vi "Real_Time_Main.vi"() -> ()   [LabVIEW 2020]
uses:
  control/uart_data.ctl
  control/logging_data.ctl
  control/system_monitoring_data.ctl
  Host/control/host_data.ctl
  <vilib>/Analysis/baseanly.llb/Mean (DBL).vi
  ae3b70e6-cfa7-4b88-a663-fdf942523340.vi
  <vilib>/Instr/_visa.llb/VISA Configure Serial Port (Instr).vi
  <vilib>/FPGAPlugInAG/cRIO-9030/niLvFpga_Open_cRIO-9030.vi
  <vilib>/rvi/interface/common/dynamic/niFpgaDynamicAddResources.vi
  <vilib>/FPGAPlugInAG/Dynamic/niLvFpga_Reset_Dynamic.vi
  <vilib>/FPGAPlugInAG/Dynamic/niLvFpga_Run_Dynamic.vi
  <vilib>/Utility/error.llb/Error Cluster From Error Code.vi
  <vilib>/rvi/errors/niLvFpgaAdjustHostInterfaceError.vi
  <vilib>/FPGAPlugInAG/Dynamic/niLvFpga_Close_Dynamic.vi
  <vilib>/rvi/interface/nirviOpenFPGA/nirviOpenFPGA.xnode
  FPGA/build/excavatorsimulat_FPGATarget_FPGAMain_YO9VNoECHsQ.lvbitx
  <vilib>/rvi/interface/nirviMethod/nirviMethod.xnode
  <vilib>/rvi/interface/nirviReadWriteControl/nirviReadWriteControl.xnode
  <vilib>/rvi/interface/nirviCloseFPGA/nirviCloseFPGA.xnode
  <vilib>/rvi/interface/Simulation/niFpgaSimulationCallBeginRW.vi
  NiFpgaLv.dll
  <vilib>/NI_Real-Time Target Support.lvlib
  <vilib>/Analysis/NI_AALBase.lvlib
  <vilib>/xnet/xnet.llb/XNET Read (Signal Single-point).vi
  <vilib>/xnet/xnet.llb/XNET Create Session (Signal Input Single-point).vi
  <vilib>/ptbypt/NI_PtbyPt.lvlib
panel:
  out "valve_duty":dbl[](array[numeric])
  out "logging_variable":T1
  out "uart_data":T2
  # "real time system not include user interface"
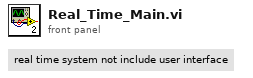
[diagram p1: front panel]
types:
  T1 = typedef "logging_data.ctl" = cluster{"time(sec)":dbl, "boom_valve_pwm":dbl, "arm_valve_pwm":dbl, "bucket_valve_pwm":dbl, "boom_angle":dbl, "arm_angle":dbl, "bucket_angle":dbl, "x_aixs_position":i32, "z_aixs_position":i32}
  T2 = typedef "uart_data.ctl" = cluster{"boom_angle":dbl, "arm_angle":dbl, "bucket_angle":dbl, "x_aixs_position":i32, "z_aixs_position":i32}
  T3 = typedef "system_monitoring_data.ctl" = cluster{"logging_state":bool, "rt_system_load":dbl, "rt_system_temp":dbl, "rt_system_absolute_time":string, "rt_system_elapse_time":string}
  T4 = enum16{"open", "replace", "create", "open or create", "replace or create", "replace or create with confirmation"}
  T5 = typedef "host_data.ctl" = cluster{"logging_enable":bool, "boom_up_signal":u8, "boom_down_signal":u8, "arm_up_signal":u8, "arm_down_signal":u8, "bucket_up_signal":u8, "bucket_down_signal":u8}
  T6 = typedef "NI_Real-Time Target Support.lvlib/RT CPU Load.ctl" = cluster{"Total (%)":dbl, "Time Critical (%)":dbl, "Timed Structures (%)":dbl, "High (%)":dbl, "Above Normal (%)":dbl, "Normal (%)":dbl, "Background (%)":dbl, "Idle (%)":dbl, "ISR (%)":dbl}
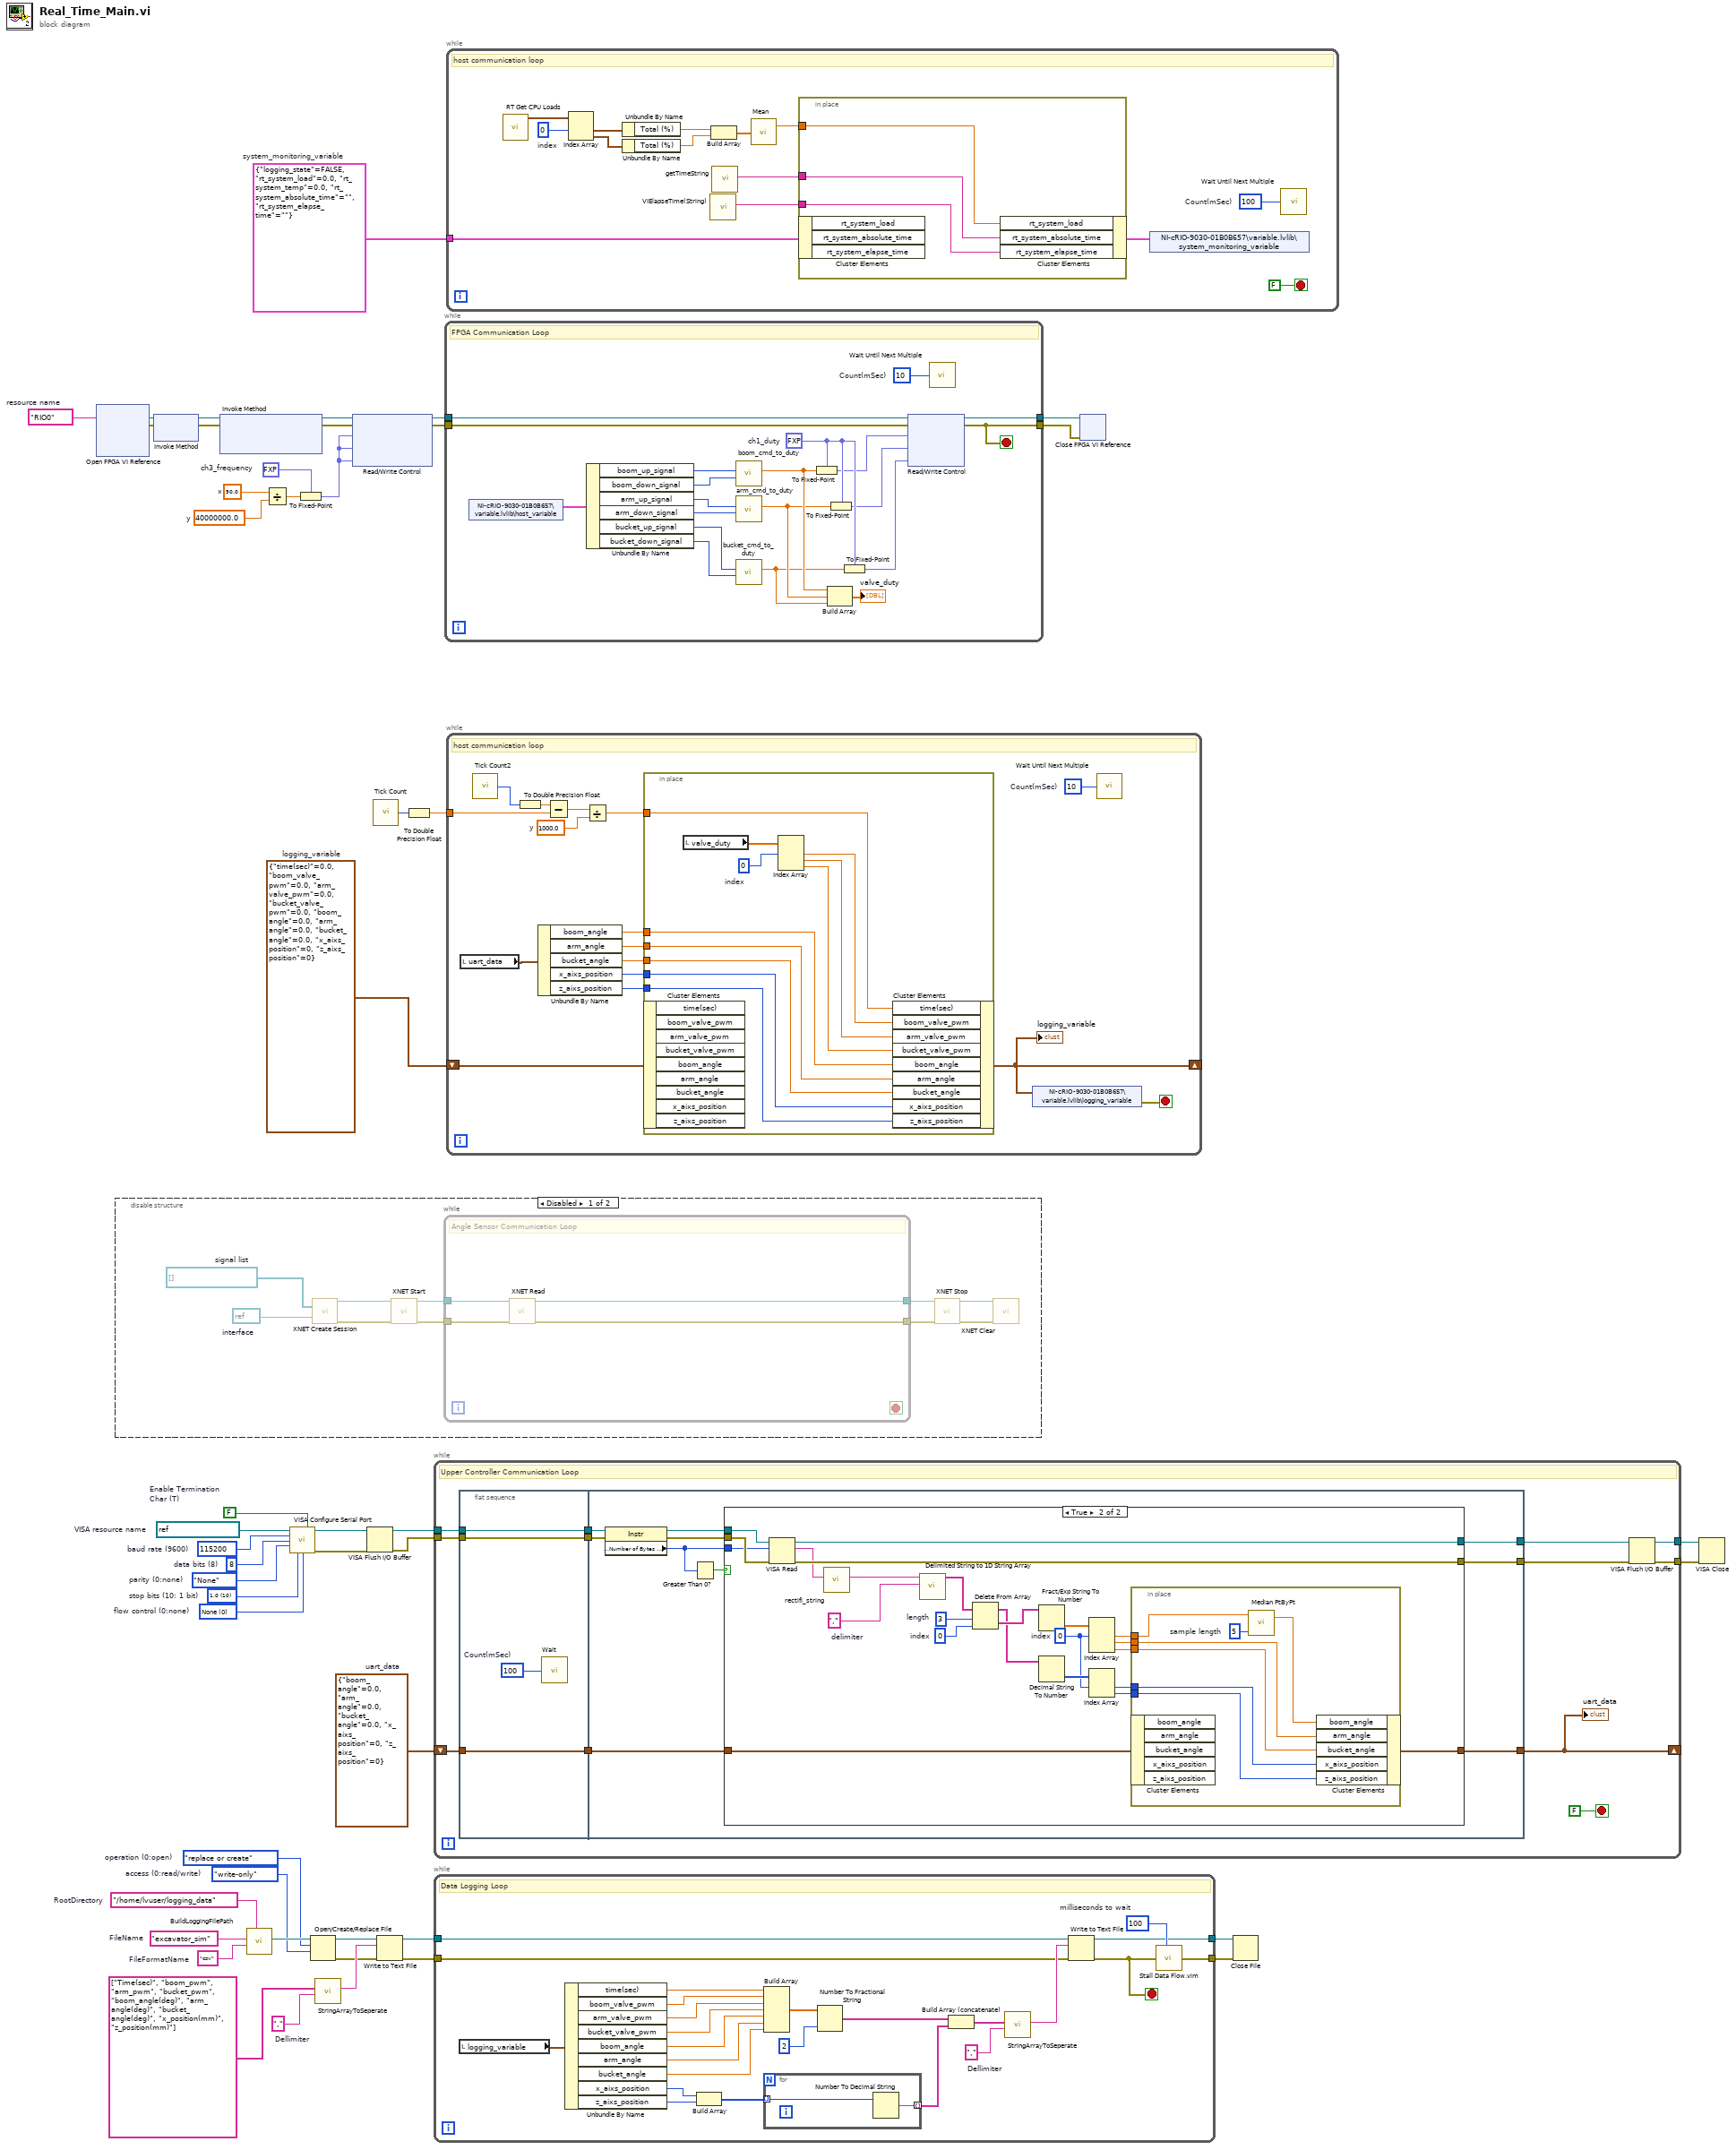
[diagram p0: block diagram]
diagram:
  w3 = T2 {"boom_angle"=0.0, "arm_angle"=0.0, "bucket_angle"=0.0, "x_aixs_position"=0, "z_aixs_position"=0}  # uart_data
  w4 = u16 0 items=["None", "XON/XOFF", "RTS/CTS", "XON/XOFF & RTS/CTS", "DTR/DSR", "XON/XOFF & DTR/DSR"]  # flow control (0:none)
  w5 = u16 10 items=["1.0"=10, "1.5"=15, "2.0"=20]  # stop bits (10: 1 bit)
  w6 = T3 {"logging_state"=FALSE, "rt_system_load"=0.0, "rt_system_temp"=0.0, "rt_system_absolute_time"="", "rt_system_elapse_time"=""}  # system_monitoring_variable
  w7 = tag "RIO0"  # resource name
  w8 = T1 {"time(sec)"=0.0, "boom_valve_pwm"=0.0, "arm_valve_pwm"=0.0, "bucket_valve_pwm"=0.0, "boom_angle"=0.0, "arm_angle"=0.0, "bucket_angle"=0.0, "x_aixs_position"=0, "z_aixs_position"=0}  # logging_variable
  w15 = 40000000.0  # y
  w16 = 50.0  # x
  w13 = fxp<+,32,0> 0.0  # ch3_frequency
  w20 = "/home/lvuser/logging_data"  # RootDirectory
  w19 = ","  # Dellimiter
  w27 = enum16{"read/write", "read-only", "write-only"}."write-only"  # access (0:read/write)
  w26 = T4."replace or create"  # operation (0:open)
  w30 = "csv"  # FileFormatName
  w31 = "excavator_sim"  # FileName
  w41 = FALSE  # Enable Termination Char (T)
  w42 = enum16{"None", "Odd", "Even", "Mark", "Space"}."None"  # parity (0:none)
  w43 = u16 8  # data bits (8)
  w44 = u32 115200  # baud rate (9600)
  w45 = refnum<visa-resource-name> "ASRL1::INSTR"  # VISA resource name
  n1 = xnode "Open FPGA VI Reference"("resource name"=w7) -> ("FPGA VI Reference Out"=w49:refnum<k20>, "error out"=w48:errorcluster)  [unwired: 1 in]
  n2 = disable-structure shown="Disabled" {
    frame Disabled {
      w58 = refnum<k21>[] []  # signal list
      w59 = refnum<k21> refnum  # interface
      n3 = call-poly <vilib>:"XNET Create Session.vi"("signal list"=w58, "interface"=w59) -> ("session out"=w57:refnum<k21>, "error out"=w56:errorcluster)  [unwired: 12 in]
      n4 = call <vilib>:"XNET Start.vi"("session in"=w57, "error in (no error)"=w56) -> ("session out"=w55:refnum<k21>, "error out"=w54:errorcluster)  [unwired: 12 in]
      n5 = while {
        tunnel: w55 -> [w64]
        tunnel: w54 -> [w63]
        tunnel: [w61] -> w53
        tunnel: [w60] -> w52
        stop <- w62 stop-if-true
        # "Angle Sensor Communication Loop"
        n6 = call-poly <vilib>:"XNET Read.vi"("session in"=w64, "error in (no error)"=w63) -> ("session out"=w61:refnum<k21>, "error out"=w60:errorcluster)  [unwired: 11 in, 1 out]
      }
      n7 = call <vilib>:"XNET Stop.vi"("session in"=w53, "error in (no error)"=w52) -> ("session out"=w51:refnum<k21>, "error out"=w50:errorcluster)  [unwired: 12 in]
      n8 = call <vilib>:"XNET Clear.vi"("session in"=w51, "error in (no error)"=w50) -> ()  [unwired: 13 in, 1 out]
    }
    frame Enabled {
    }
  }
  n9 = xnode "Invoke Method"("FPGA VI Reference In"=w49, "error in"=w48) -> ("FPGA VI Reference Out"=w47:refnum<k20>, "error out"=w46:errorcluster)
  n10 = xnode "Invoke Method"("FPGA VI Reference In"=w47, "error in"=w46) -> ("FPGA VI Reference Out"=w36:refnum<k20>, "error out"=w17:errorcluster)  [unwired: 1 in]
  n11 = call "BuildLoggingFilePath.vi"("RootDirectory"=w20, "FileFormatName"=w30, "FileName"=w31) -> ("appended path"=w32:path)  [unwired: 8 in]
  n12 = Divide(x=w16, y=w15) -> (x/y=w14:dbl)
  n13 = call-poly "VISA Configure Serial Port"("VISA resource name"=w45, "Enable Termination\nChar (T)"=w41, "baud rate (9600)"=w44, "data bits (8)"=w43, "parity (0:none)"=w42, "stop bits (10: 1 bit)"=w5, "flow control (0:none)"=w4) -> ("VISA resource name out"=w40:refnum<visa-resource-name>, "error out"=w39:errorcluster)  [unwired: 7 in]
  n14 = To Fixed-Point(fixed-point type=w13, number=w14) -> (fixed-point=w12:fxp<+,32,0>)
  n15 = Open/Create/Replace File(file path (use dialog)=w32, operation (0:open)=w26, access (0:read/write)=w27) -> (refnum out=w28:refnum<file>, error out=w29:errorcluster)  [unwired: 3 in, 1 out]
  n16 = call "StringArrayToSeperate.vi"("Delimiter"=w19, "StringArray"=string[] ["Time(sec)", "boom_pwm", "arm_pwm", "bucket_pwm", "boom_angle(deg)", "arm_angle(deg)", "bucket_angle(deg)", "x_position(mm)", "z_position(mm)"]) -> ("String"=w33:string)  [unwired: 9 in]
  n17 = xnode "Read/Write Control"("FPGA VI Reference In"=w36, "error in"=w17, "ch1_frequency"=w12, "ch2_frequency"=w12, "ch3_frequency"=w12) -> ("FPGA VI Reference Out"=w18:refnum<k20>, "error out"=w11:errorcluster)
  n18 = VISA Flush I/O Buffer(VISA resource name=w40, error in (no error)=w39) -> (VISA resource name out=w38:refnum<visa-resource-name>, error out=w37:errorcluster)  [unwired: 1 in]
  n19 = call "Tick Count"() -> ("Tick Count(mSec)"=w10:u32)
  n20 = Write to Text File(file (use dialog)=w28, text=w33, error in=w29) -> (refnum out=w25:refnum<file>, error out=w24:errorcluster)  [unwired: 1 in, 1 out]
  n21 = To Double Precision Float(number=w10) -> (double precision float=w9:dbl)
  n22 = while {
    tunnel: w38 -> [w74]
    tunnel: w37 -> [w72]
    shift-right: [w69] -> _
    shift-left: w3 -> [w70]
    tunnel: [w67] -> w2
    tunnel: [w65] -> w1
    stop <- FALSE stop-if-true
    # "Upper Controller Communication Loop"
    n23 = flat-sequence {
      tunnel: [w79] -> w75
      tunnel: w74 -> [w79]
      tunnel: [w78] -> w73
      tunnel: w72 -> [w78]
      tunnel: [w77] -> w71
      tunnel: w70 -> [w77]
      tunnel: w75 -> [w90]
      tunnel: w73 -> [w89]
      tunnel: w71 -> [w85]
      tunnel: [w86] -> w68
      tunnel: [w84] -> w69
      tunnel: [w81] -> w66
      frame #0 {
        w80 = u32 100  # Count(mSec)
        n24 = call "Wait"("Count(mSec)"=w80) -> ()  [unwired: 1 out]
      }
      frame #1 {
        n25 = property class="Instr"(reference=w90, error in=w89) -> (reference out=w88:refnum<visa-resource-name>, error out=w87:errorcluster, "Serial Settings:Number of Bytes at Serial Port"=w82:u32)
        n26 = Greater Than 0?(x=w82) -> (x > 0?=w83:bool)
        n27 = case shown="True" w83 {
          tunnel: w88 -> [w92 w116]
          tunnel: w82 -> [_ w96]
          tunnel: w87 -> [w91 w115]
          tunnel: [w92 w113] -> w86
          tunnel: [w91 w112] -> w81
          tunnel: w85 -> [w93 w111]
          tunnel: [w93 w110] -> w84
          frame False {
          }
          frame True {
            w103 = 0  # index
            w104 = 3  # length
            w99 = 0  # index
            w114 = ","  # delimiter
            n28 = VISA Read(VISA resource name=w116, byte count=w96, error in (no error)=w115) -> (VISA resource name out=w113:refnum<visa-resource-name>, read buffer=w95:string, error out=w112:errorcluster)  [unwired: 1 out]
            n29 = call "rectifi_string.vi"("input"=w95) -> ("output"=w94:string)  [unwired: 10 in]
            n30 = call <vilib>:"Delimited String to 1D String Array.vi"("delimiter"=w114, "delimited string"=w94) -> ("string array"=w105:string[])  [unwired: 9 in]
            n31 = Delete From Array "Delete From Array"(array=w105, length=w104, index=w103) -> (deleted portion=w98:string[], array with subset deleted=w97:string[])
            n32 = Fract/Exp String To Number(string=w98) -> (number=w109:dbl[])  [unwired: 3 in, 1 out]
            n33 = Decimal String To Number(string=w97) -> (number=w102:i32[])  [unwired: 2 in, 1 out]
            n34 = Index Array(array=w109, index #1=w99) -> (element #1=w108:dbl, element #2=w107:dbl, element #3=w106:dbl)  [unwired: 2 in]
            n35 = Index Array(array=w102, index #1=w99) -> (element #1=w101:i32, element #2=w100:i32)  [unwired: 1 in]
            n36 = in-place {
              in-place-border: w108 -> [w118]
              in-place-border: w107 -> [w123]
              in-place-border: w106 -> [w122]
              in-place-border: w101 -> [w121]
              in-place-border: w100 -> [w120]
              w119 = 5  # sample length
              n37 = in-place-cluster #1(w111) -> ()  [unwired: 5 out]
              n38 = call <vilib>:"Median PtByPt.vi"("sample length"=w119, "x"=w118) -> ("median"=w117:dbl)  [unwired: 2 in, 1 out]
              n39 = in-place-cluster #1("boom_angle"=w117, "arm_angle"=w123, "bucket_angle"=w122, "x_aixs_position"=w121, "z_aixs_position"=w120) -> (w110:T2)
            }
          }
        }
      }
    }
    n40 = VISA Flush I/O Buffer(VISA resource name=w68, error in (no error)=w66) -> (VISA resource name out=w67:refnum<visa-resource-name>, error out=w65:errorcluster)  [unwired: 1 in]
    "uart_data" <- w69
  }
  n41 = while {
    tunnel: w25 -> [w143]
    tunnel: w24 -> [w142]
    tunnel: [w141] -> w23
    tunnel: [w140] -> w22
    stop <- w145 stop-if-true
    w139 = ","  # Dellimiter
    w144 = u32 100  # milliseconds to wait
    # "Data Logging Loop"
    n42 = local read "logging_variable"() -> (w138:T1)
    n43 = Unbundle By Name(w138) -> ("time(sec)"=w137:dbl, "boom_valve_pwm"=w136:dbl, "arm_valve_pwm"=w135:dbl, "bucket_valve_pwm"=w134:dbl, "boom_angle"=w133:dbl, "arm_angle"=w132:dbl, "bucket_angle"=w131:dbl, "x_aixs_position"=w129:i32, "z_aixs_position"=w128:i32)
    n44 = Build Array(w129, w128) -> (w127:i32[])
    n45 = for {
      tunnel: w127 -> [w149] mode=indexing
      tunnel: [w148] -> w125 mode=indexing
      n46 = Number To Decimal String(number=w149) -> (decimal integer string=w148:string)  [unwired: 1 in]
    }
    n47 = Build Array(w137, w136, w135, w134, w133, w132, w131) -> (w130:dbl[])
    n48 = Number To Fractional String(number=w130, precision (6)=i16 2) -> (F-format string=w126:string[])  [unwired: 2 in]
    n49 = Build Array (concatenate)(w126, w125) -> (w124:string[])
    n50 = call "StringArrayToSeperate.vi"("Delimiter"=w139, "StringArray"=w124) -> ("String"=w147:string)  [unwired: 9 in]
    n51 = Write to Text File(file (use dialog)=w143, text=w147, error in=w142) -> (refnum out=w141:refnum<file>, error out=w145:errorcluster)  [unwired: 1 in, 1 out]
    n52 = call "Stall Data Flow.vim"("value in"=w145, "milliseconds to wait"=w144) -> ("value out"=w140:errorcluster)  [unwired: 1 out]
  }
  n53 = while {
    tunnel: [w169] -> w35
    tunnel: [w161] -> w34
    tunnel: w18 -> [w168]
    tunnel: w11 -> [w167]
    stop <- w161 stop-if-true
    w165 = fxp<+,32,0> 0.0  # ch1_duty
    w166 = u32 10  # Count(mSec)
    # "FPGA Communication Loop"
    n54 = shared-variable "NI-cRIO-9030-01B0B657\\variable.lvlib\\host_variable"() -> (w150:T5)  [unwired: 1 in, 1 out]
    n55 = Unbundle By Name(w150) -> ("boom_up_signal"=w160:u8, "boom_down_signal"=w159:u8, "arm_up_signal"=w158:u8, "arm_down_signal"=w157:u8, "bucket_up_signal"=w156:u8, "bucket_down_signal"=w155:u8)
    n56 = call "boom_cmd_to_duty.vi"("boom_down_signal"=w159, "boom_up_signal"=w160) -> ("duty"=w154:dbl)  [unwired: 9 in]
    n57 = call "arm_cmd_to_duty.vi"("arm_down_signal"=w157, "arm_up_signal"=w158) -> ("duty"=w153:dbl)  [unwired: 9 in]
    n58 = call "bucket_cmd_to_duty.vi"("bucket_down_signal"=w155, "bucket_up_signal"=w156) -> ("duty"=w152:dbl)  [unwired: 9 in]
    n59 = To Fixed-Point(fixed-point type=w165, number=w154) -> (fixed-point=w164:fxp<+,32,0>)
    n60 = Build Array(w154, w153, w152) -> (→"valve_duty":dbl[])
    n61 = To Fixed-Point(fixed-point type=w165, number=w153) -> (fixed-point=w163:fxp<+,32,0>)
    n62 = To Fixed-Point(fixed-point type=w165, number=w152) -> (fixed-point=w162:fxp<+,32,0>)
    n63 = xnode "Read/Write Control"("FPGA VI Reference In"=w168, "error in"=w167, "ch1_duty"=w164, "ch2_duty"=w163, "ch3_duty"=w162) -> ("FPGA VI Reference Out"=w169:refnum<k20>, "error out"=w161:errorcluster)
    n64 = call "Wait Until Next Multiple"("Count(mSec)"=w166) -> ()  [unwired: 1 out]
  }
  n65 = while {
    tunnel: w6 -> [w174]
    stop <- FALSE stop-if-true
    w180 = 0  # index
    w182 = u32 100  # Count(mSec)
    # "host communication loop"
    n66 = call <vilib>:"RT Get CPU Loads.vi"() -> ("CPU loads"=w181:T6[])  [unwired: 10 in, 1 out]
    n67 = Index Array(array=w181, index #1=w180) -> (element #1=w179:T6, element #2=w178:T6)  [unwired: 1 in]
    n68 = Unbundle By Name(w179) -> ("Total (%)"=w177:dbl)
    n69 = Unbundle By Name(w178) -> ("Total (%)"=w176:dbl)
    n70 = call "VIElapseTime(String).vi"() -> ("ElapseTime"=w170:string)  [unwired: 11 in]
    n71 = Build Array(w177, w176) -> (w175:dbl[])
    n72 = call "getTimeString.vi"() -> ("getTime"=w171:string)  [unwired: 11 in]
    n73 = call-poly <vilib>:"Mean.vi"("X"=w175) -> ("mean"=w173:dbl)  [unwired: 1 out]
    n74 = in-place {
      in-place-border: w173 -> [w186]
      in-place-border: w171 -> [w185]
      in-place-border: w170 -> [w184]
      n75 = in-place-cluster #2(w174) -> ()  [unwired: 3 out]
      n76 = in-place-cluster #2("rt_system_load"=w186, "rt_system_absolute_time"=w185, "rt_system_elapse_time"=w184) -> (w172:T3)
    }
    n77 = shared-variable "NI-cRIO-9030-01B0B657\\variable.lvlib\\system_monitoring_variable"(w172) -> ()  [unwired: 1 in, 1 out]
    n78 = call "Wait Until Next Multiple"("Count(mSec)"=w182) -> ()  [unwired: 1 out]
  }
  n79 = while {
    tunnel: w9 -> [w200]
    shift-right: [w193] -> _
    shift-left: w8 -> [w197]
    stop <- w198 stop-if-true
    w195 = 1000.0  # y
    w202 = u32 10  # Count(mSec)
    # "host communication loop"
    n80 = local read "uart_data"() -> (w192:T2)
    n81 = call "Tick Count2"() -> ("Tick Count(mSec)"=w201:u32)
    n82 = To Double Precision Float(number=w201) -> (double precision float=w199:dbl)
    n83 = Unbundle By Name(w192) -> ("boom_angle"=w191:dbl, "arm_angle"=w190:dbl, "bucket_angle"=w189:dbl, "x_aixs_position"=w188:i32, "z_aixs_position"=w187:i32)
    n84 = Subtract(x=w199, y=w200) -> (x-y=w196:dbl)
    n85 = Divide(x=w196, y=w195) -> (x/y=w194:dbl)
    n86 = in-place {
      in-place-border: w194 -> [w213]
      in-place-border: w191 -> [w212]
      in-place-border: w190 -> [w211]
      in-place-border: w189 -> [w210]
      in-place-border: w188 -> [w209]
      in-place-border: w187 -> [w208]
      w203 = 0  # index
      n87 = in-place-cluster #3(w197) -> ()  [unwired: 9 out]
      n88 = local read "valve_duty"() -> (w207:dbl[])
      n89 = Index Array(array=w207, index #1=w203) -> (element #1=w206:dbl, element #2=w205:dbl, element #3=w204:dbl)  [unwired: 2 in]
      n90 = in-place-cluster #3("time(sec)"=w213, "boom_valve_pwm"=w206, "arm_valve_pwm"=w205, "bucket_valve_pwm"=w204, "boom_angle"=w212, "arm_angle"=w211, "bucket_angle"=w210, "x_aixs_position"=w209, "z_aixs_position"=w208) -> (w193:T1)
    }
    "logging_variable" <- w193
    n91 = shared-variable "NI-cRIO-9030-01B0B657\\variable.lvlib\\logging_variable"(w193) -> (error out=w198:errorcluster)  [unwired: 1 in]
    n92 = call "Wait Until Next Multiple"("Count(mSec)"=w202) -> ()  [unwired: 1 out]
  }
  n93 = xnode "Close FPGA VI Reference"("FPGA VI Reference In"=w35, "error in"=w34) -> ()  [unwired: 1 out]
  n94 = Close File(refnum=w23, error in=w22) -> ()  [unwired: 2 out]
  n95 = VISA Close(VISA resource name=w2, error in (no error)=w1) -> ()  [unwired: 1 out]
